vi "Vision Code_3.vi"(0 "Image In":T1, 1 "Image Dst":T1, 7 "error in":errorcluster) -> (20 "Image Out":T1, 27 "error out":errorcluster)   [LabVIEW 2014]
doc: "Creates, edits, and runs vision algorithms using NI Vision Assistant.\n\nWhen you place this Express VI on the block diagram, NI Vision Assistant launches. Create an algorithm using the Vision Assistant processing functions. After you create an algorithm, you can select the controls and indicators that you want to be able to programmatically set in LabVIEW. Double-click the Vision Assistant Express VI to edit the algorithm."
uses:
  <vilib>/vision/Image Controls.llb/IMAQ Image.ctl
  <vilib>/vision/NI_Vision_Development_Module.lvlib
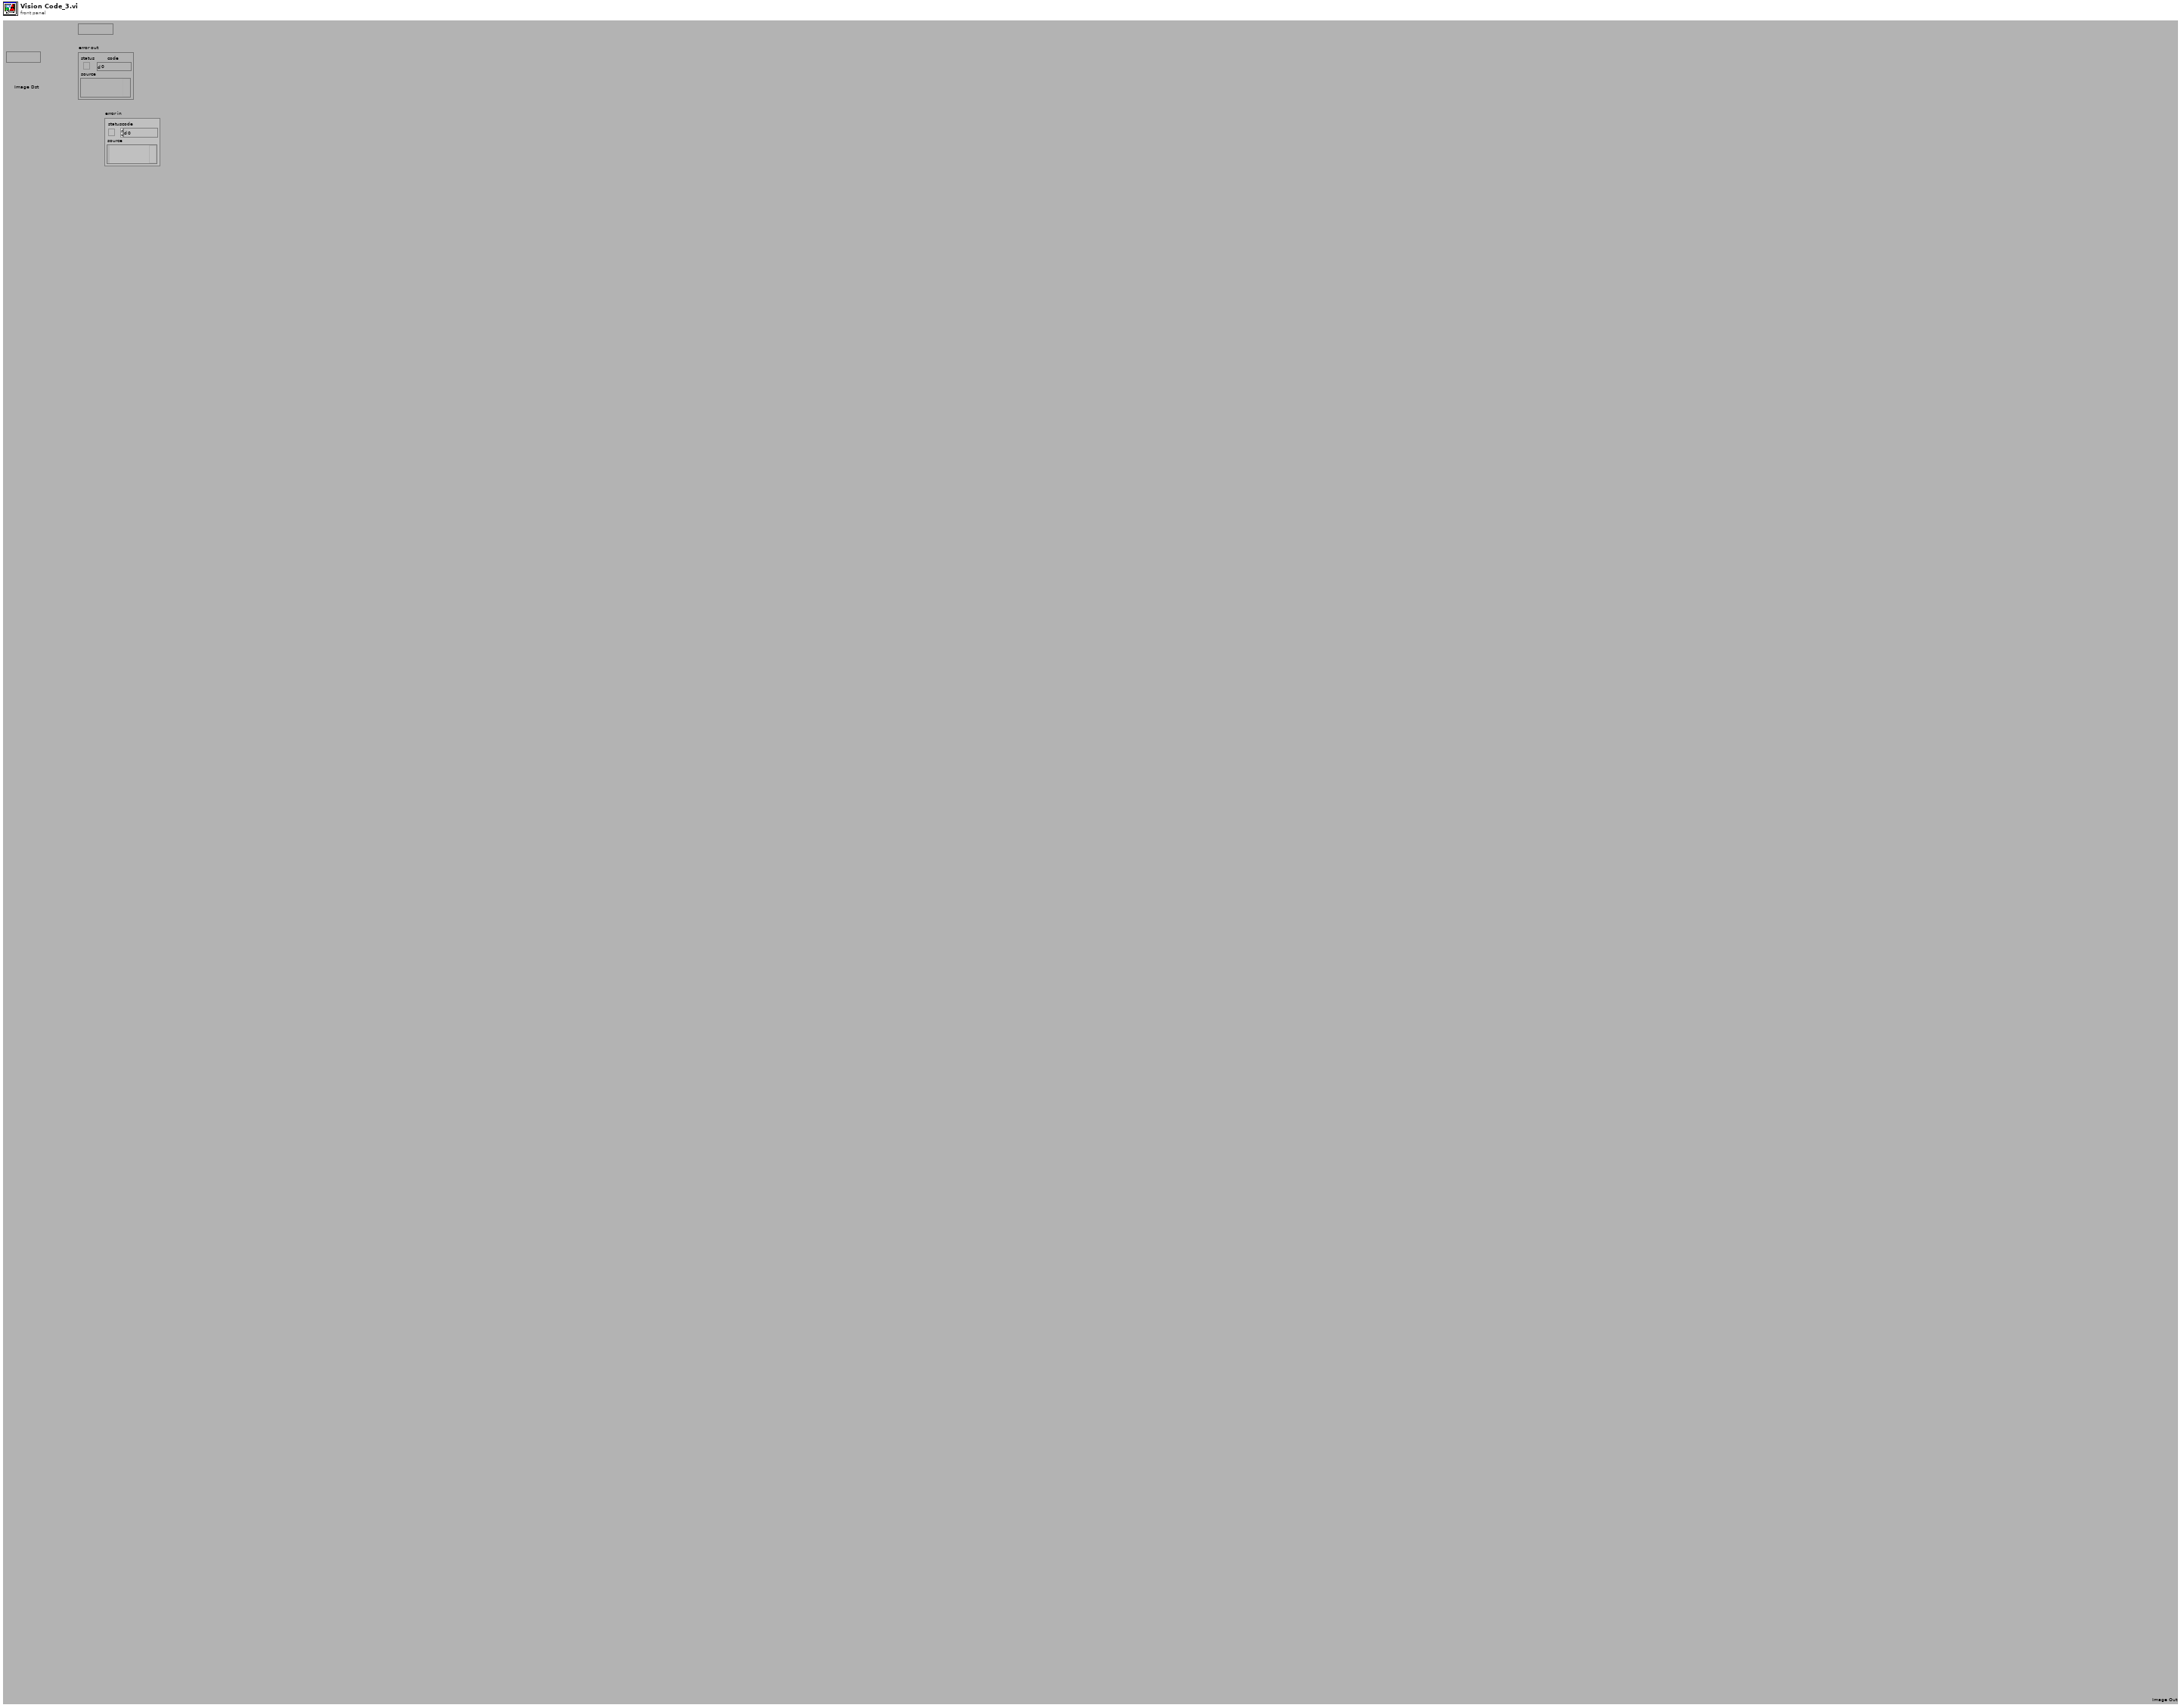
[diagram p1: front panel]
types:
  T1 = typedef "IMAQ Image.ctl" = refnum<image>
  T2 = cluster{"Contrast":i32, "Filter width":i32, "Steepness":i32, "Subsampling Ratio":u32, "Show Search Area":bool, "Show Search Lines":bool, "Show Edges Found":bool, "Show Result":bool}
  T3 = cluster{"Global Rectangle":i32[], "Contours":cluster{"ID":enum32{"External", "Internal"}, "Type":u32, "Coordinates":i32[]}[]}
  T4 = enum32{"AutoM", "Close", "Dilate", "Erode", "Gradient", "Gradient out", "Gradient in", "Hit miss", "Open", "PClose", "POpen", "Thick", "Thin"}
  T5 = typedef "Image Type" = u32
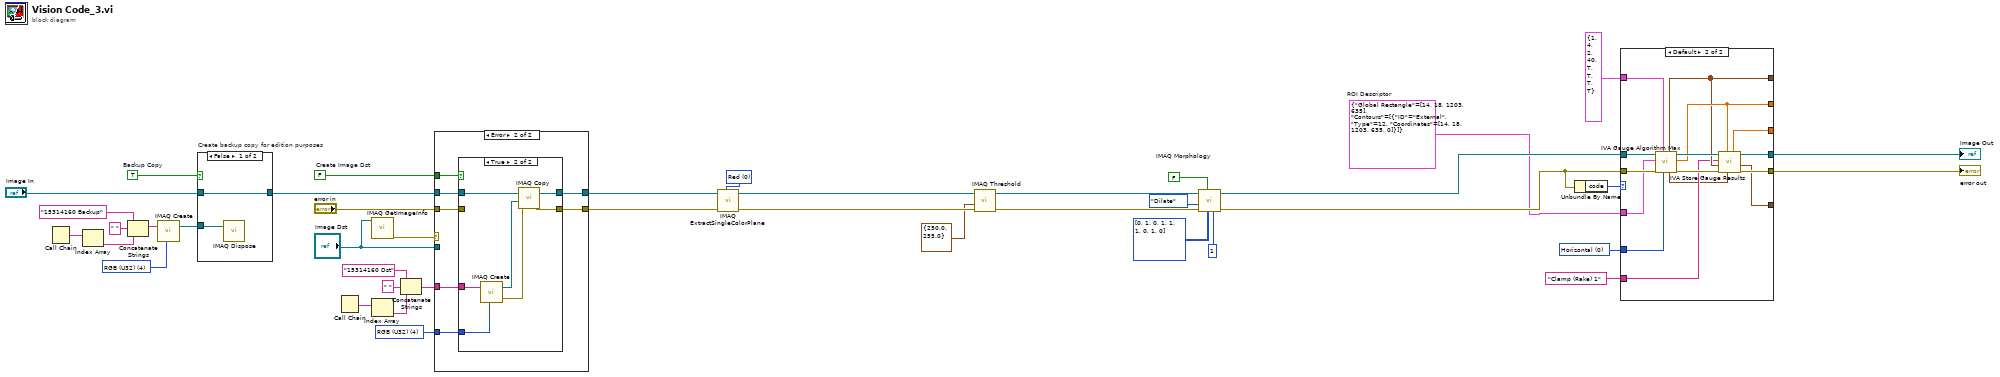
[diagram p0: block diagram]
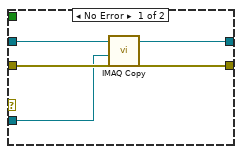
[diagram p3: hidden frame]
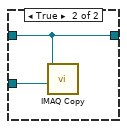
[diagram p5: hidden frame]
diagram:
  w6 = u32 0 items=["Horizontal", "Vertical"] ("Scanning axis")
  w5 = T3 {"Global Rectangle"=[14, 18, 1203, 635], "Contours"=[{"ID"=enum."External", "Type"=12, "Coordinates"=[14, 18, 1203, 635, 0]}]}  # ROI Descriptor
  w20 = 0 items=["Red", "Green", "Blue", "Hue", "Saturation", "Luminance", "Value", "Intensity"] ("Color Plane")
  w21 = T5 4 items=["Grayscale (U8)", "Grayscale (I16)", "Grayscale (SGL)", "Complex (CSG)", "RGB (U32)", "HSL (U32)", "RGB (U64)", "Grayscale (U16)"] ("Image Dst Type")
  w22 = T5 4 items=["Grayscale (U8)", "Grayscale (I16)", "Grayscale (SGL)", "Complex (CSG)", "RGB (U32)", "HSL (U32)", "RGB (U64)", "Grayscale (U16)"] ("Image Type")
  w41 = TRUE  # Backup Copy
  w34 = FALSE  # Create Image Dst
  n1 = Call Chain() -> (call chain=w28:string[])
  n2 = Index Array(array=w28) -> (element=w27:string)  [unwired: 1 in]
  n3 = Concatenate Strings("15314160 Backup" ("Backup Image Name"), " ", w27) -> (w24:string)
  n4 = call "IMAQ Create"("Image Name"=w24, "Image Type"=w22) -> ("New Image"=w23:T1)  [unwired: 2 in, 2 out]
  n5 = case "Create backup copy for edition purposes" shown="False" w41 {
    tunnel: [w43 w45] -> w37
    tunnel: "Image In" -> [w43 w45]
    tunnel: w23 -> [w42 w44]
    frame False {
      n6 = call "IMAQ Dispose"("Image"=w42) -> ()  [unwired: 2 in, 4 out]
    }
    frame True {
      n7 = call "IMAQ Copy"("Image Dst"=w44, "Image Src"=w45) -> ()  [unwired: 1 in, 5 out]
    }
  }
  n8 = Call Chain() -> (call chain=w33:string[])
  n9 = call "IMAQ GetImageInfo"("Image"="Image Dst") -> ("error out"=w39:errorcluster)  [unwired: 1 in, 9 out]
  n10 = Index Array(array=w33) -> (element=w31:string)  [unwired: 1 in]
  n11 = Concatenate Strings("15314160 Dst" ("Image Dst Name"), " ", w31) -> (w29:string)
  n12 = case shown="Error" w39 {
    tunnel: [w50 w54] -> w19
    tunnel: [w49 w53] -> w35
    tunnel: w37 -> [w48 w55]
    tunnel: "error in" -> [w47 w51]
    tunnel: "Image Dst" -> [w46 _]
    tunnel: w29 -> [_ w57]
    tunnel: w21 -> [_ w56]
    tunnel: w34 -> [_ w52]
    frame No Error {
      n13 = call "IMAQ Copy"("error in (no error)"=w47, "Image Dst"=w46, "Image Src"=w48) -> ("error out"=w49:errorcluster, "Image Dst Out"=w50:T1)  [unwired: 3 out]
    }
    frame Error {
      n14 = case shown="True" w52 {
        tunnel: w57 -> [_ w66]
        tunnel: w56 -> [_ w65]
        tunnel: w55 -> [w59 w63]
        tunnel: [w59 w62] -> w54
        tunnel: [w58 w61] -> w53
        tunnel: w51 -> [w58 _]
        frame False {
        }
        frame True {
          n15 = call "IMAQ Create"("Image Name"=w66, "Image Type"=w65) -> ("New Image"=w64:T1, "error out"=w60:errorcluster)  [unwired: 2 in, 1 out]
          n16 = call "IMAQ Copy"("error in (no error)"=w60, "Image Dst"=w64, "Image Src"=w63) -> ("error out"=w61:errorcluster, "Image Dst Out"=w62:T1)  [unwired: 3 out]
        }
      }
    }
  }
  n17 = call "IMAQ ExtractSingleColorPlane"("Color Plane"=w20, "error in (no error)"=w35, "Image Src"=w19) -> ("error out"=w18:errorcluster, "Image Dst Out"=w16:T1)  [unwired: 1 in, 6 out]
  n18 = call "IMAQ Threshold"("error in (no error)"=w18, "Range"=cluster{"Lower value":sgl, "Upper value":sgl} {"Lower value"=250.0, "Upper value"=255.0}, "Image Src"=w16) -> ("error out"=w15:errorcluster, "Image Dst Out"=w10:T1)  [unwired: 3 in, 4 out]
  n19 = call "IMAQ Morphology"("Number of iterations (1)"=1, "Structuring Element"=i32[][] [[0, 1, 0], [1, 1, 1], [0, 1, 0]], "Square/Hexa (Square)"=FALSE, "error in (no error)"=w15, "Operation"=T4."Dilate", "Image Src"=w10) -> ("error out"=w9:errorcluster, "Image Dst Out"=w8:T1)  [unwired: 1 in, 3 out]
  n20 = Unbundle By Name(w9) -> ("code"=w3:i32)
  n21 = case shown="Default" w3 {
    tunnel: w8 -> [w67 w82]
    tunnel: w9 -> [_ w81]
    tunnel: T2 {"Contrast"=1, "Filter width"=4, "Steepness"=2, "Subsampling Ratio"=40, "Show Search Area"=TRUE, "Show Search Lines"=TRUE, "Show Edges Found"=TRUE, "Show Result"=TRUE} ("Settings") -> [_ w80]
    tunnel: w6 -> [_ w79]
    tunnel: w5 -> [_ w78]
    tunnel: [w67 w76] -> w1
    tunnel: [_ w74] -> w4
    tunnel: [_ w73] -> _
    tunnel: [_ w72] -> _
    tunnel: [_ w71] -> _
    tunnel: [_ w70] -> _
    tunnel: "Clamp (Rake) 1" ("Step Name") -> [_ w69]
    frame -1074396199, -1074396198 {
      # "Discard Coordinate System Error"
    }
    frame Default {
      n22 = call <vilib>:"IVA Gauge Algorithm Max.vi"("Scanning axis"=w79, "Settings"=w80, "error in (no error)"=w81, "ROI Descriptor"=w78, "Image"=w82) -> ("error out"=w75:errorcluster, "Distance"=w73:sgl, "Image Out"=w77:T1, "Distance Points"=w68:cluster{"X":sgl, "Y":sgl}[], "Points of Contact"=w72:cluster{"X":sgl, "Y":sgl}[])  [unwired: 1 in, 1 out]
      n23 = call <vilib>:"IVA Store Gauge Results.vi"("Distance Points"=w68, "Distance"=w73, "error in (no error)"=w75, "Points of Contact"=w72, "Step Name"=w69, "Image in"=w77) -> ("error out"=w74:errorcluster, "Points of Contact (calibrated)"=w70:cluster{"X":sgl, "Y":sgl}[], "Image dup"=w76:T1, "Distance (calibrated)"=w71:sgl)  [unwired: 2 out]
    }
  }
  "error out" <- w4
  "Image Out" <- w1
